vi "LightingSystem_Create.vi"(0 "reference in":refnum<class "LightingSystem.lvclass">, 2 "Rooms":T1, 5 "Error In":errorcluster) -> (14 "reference out":refnum<class "LightingSystem.lvclass">, 19 "Error Out":errorcluster)   [LabVIEW 2024, in "LightingSystem.lvclass"]
uses:
  LightingSystem.lvclass
  LightingSystem.lvclass/LightingSystem.ctl
  House/Room_class/Room.lvclass
  Type Defs/Rooms Cluster Array.ctl
panel:
  # "Connector Pane"
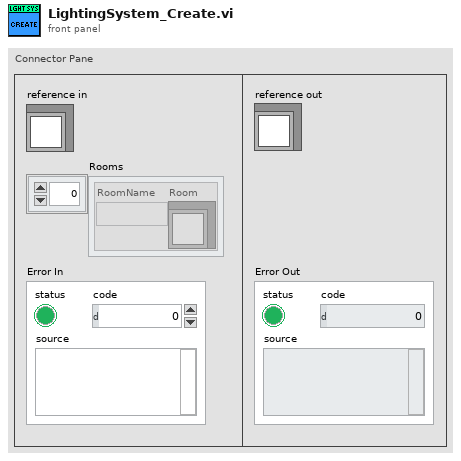
[diagram p1: front panel]
types:
  T1 = typedef "Rooms Cluster Array.ctl" = cluster{"RoomName":string, "Room":refnum<class "Room.lvclass">}[]
  T2 = typedef "LightingSystem.lvclass/ObjectAttributes.ctl" = cluster{"Rooms":T3}
  T3 = typedef "Rooms Map.ctl" = map{string, refnum<class "Room.lvclass">}
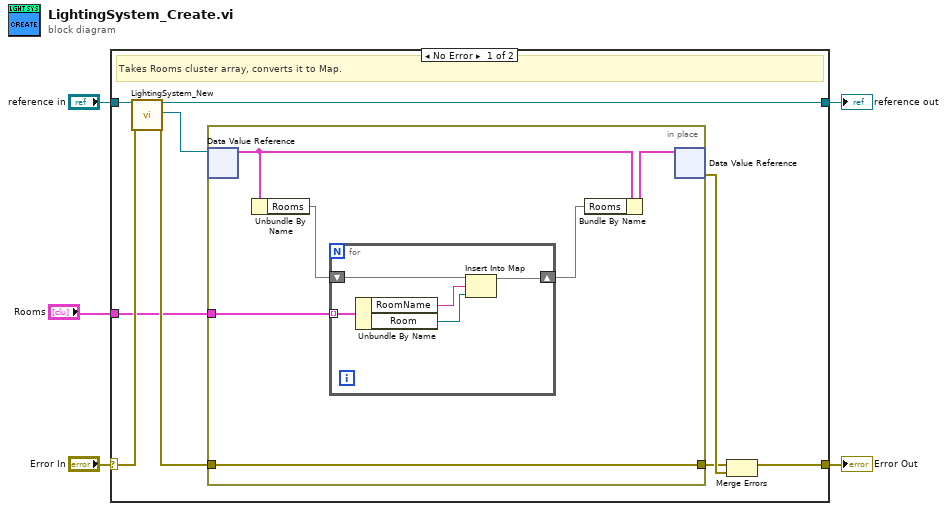
[diagram p0: block diagram]
diagram:
  n1 = case shown="No Error" "Error In" {
    selector: "Error In" -> [w13 w27]
    tunnel: [w10 w27] -> w4
    tunnel: "reference in" -> [w14 w26]
    tunnel: [w12 w26] -> w2
    tunnel: "Rooms" -> [w6 _]
    frame No Error {
      # "Takes Rooms cluster array, converts it to Map."
      n2 = call "LightingSystem_New.vi"("reference in"=w14, "Error In"=w13) -> ("reference out"=w12:refnum<class "LightingSystem.lvclass">, "DVRRefOut"=w9:refnum<data-value>, "Error Out"=w8:errorcluster)  [unwired: 14 in, 1 out]
      n3 = in-place {
        in-place-border: w8 -> [w18]
        in-place-border: [w18] -> w7
        in-place-border: w6 -> [w15]
        n4 = in-place-dvr #1(w9) -> (w19:T2)  [unwired: 1 out]
        n5 = Unbundle By Name(w19) -> ("Rooms"=w17:T3)
        n6 = for {
          shift-right: [w24] -> w16
          shift-left: w17 -> [w25]
          tunnel: w15 -> [w23] mode=indexing
          n7 = Unbundle By Name(w23) -> ("RoomName"=w22:string, "Room"=w21:refnum<class "Room.lvclass">)
          n8 = Insert Into Map(map in=w25, key=w22, value=w21) -> (map out=w24:T3)  [unwired: 2 out]
        }
        n9 = Bundle By Name(cluster=w19, "Rooms"=w16) -> (w20:T2)
        n10 = in-place-dvr #1(w20) -> (w11:errorcluster)  [unwired: 1 out]
      }
      n11 = Merge Errors(w7, w11) -> (w10:errorcluster)
    }
    frame Error {
      # "VI-TechBaseTemplate_Simple_6x8x6"
    }
  }
  "Error Out" <- w4
  "reference out" <- w2
